vi "subGetComponentReferencesRefs.vi"(8 "error in (no error)":errorcluster, 11 "Refnum in":refnum<k20>) -> (0 "error out":errorcluster, 1 "Concession Node Ref out":refnum<k20>, 2 "Allow Node Ref out":refnum<k20>, 3 "Refnum out":refnum<k20>)   [LabVIEW 2020, in "DefaultExtensions.lvlib" / "CDefaultRuleFileParser.lvclass"]
uses:
  CDefaultRuleFileParser.lvclass
  <vilib>/xml/NI_XML.lvlib
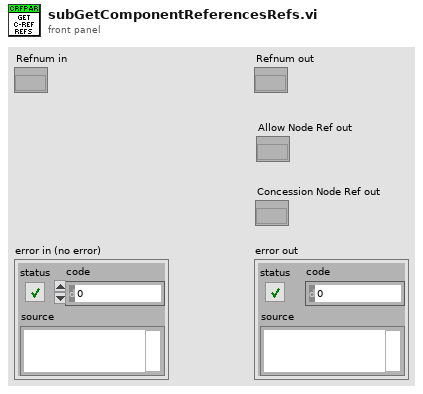
[diagram p1: front panel]
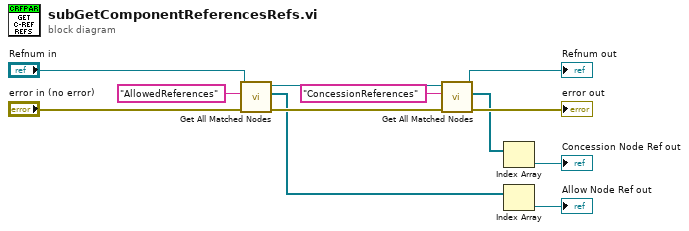
[diagram p0: block diagram]
diagram:
  n1 = call <vilib>:"Get All Matched Nodes.vi"("error in (no error)"="error in (no error)", "XPath expression"="AllowedReferences", "node in"="Refnum in") -> ("error out"=w9:errorcluster, "node result array"=w4:refnum<k20>[], "node out"=w8:refnum<k20>)  [unwired: 6 in]
  "error out" <- w9
  n2 = call <vilib>:"Get All Matched Nodes.vi"("error in (no error)"=w9, "XPath expression"="ConcessionReferences", "node in"=w8) -> ("node result array"=w6:refnum<k20>[], "node out"=→"Refnum out":refnum<k20>)  [unwired: 6 in, 1 out]
  n3 = Index Array(array=w6) -> (element=→"Concession Node Ref out":refnum<k20>)  [unwired: 1 in]
  n4 = Index Array(array=w4) -> (element=→"Allow Node Ref out":refnum<k20>)  [unwired: 1 in]
